vi "Practica3_led.vi"() -> ()   [LabVIEW 2015]
uses:
  <vilib>/LabVIEW Interface for Arduino/Type Defs/Pin Mode.ctl
  <vilib>/LabVIEW Interface for Arduino/LabVIEW Interface for Arduino.lvlib
panel:
  in  "Encendido":dbl format="%#.4g"
  in  "Apagado":dbl
  in  "stop":bool
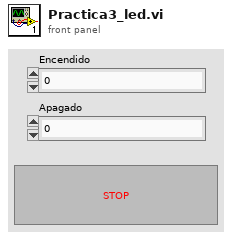
[diagram p1: front panel]
types:
  T1 = typedef "LabVIEW Interface for Arduino.lvlib/Pin Mode.ctl" = enum8{"Input", "Output"}
  T2 = typedef "LabVIEW Interface for Arduino.lvlib/Arduino Resource.ctl" = cluster{"VISA resource":refnum<visa-resource-name>, "Board Type":T3, "Connection Type":enum8{"USB / Serial"}, "Bytes Per Packet (15)":u8}
  T3 = typedef "LabVIEW Interface for Arduino.lvlib/Board Type.ctl" = enum16{"Uno", "Dimuelanove w/Atmega 328", "Mega 2560"}
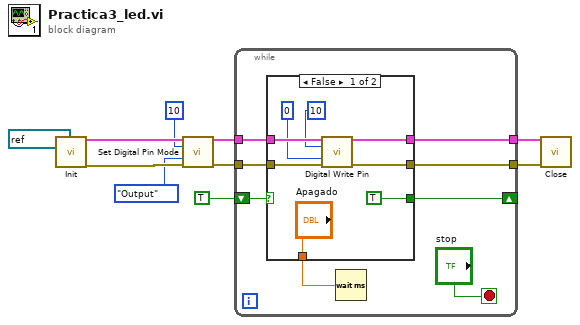
[diagram p0: block diagram]
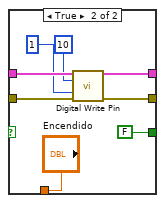
[diagram p2: hidden frame]
diagram:
  n1 = call <vilib>:"Init.vi"("VISA resource"=refnum<visa-resource-name> "COM4") -> ("Arduino Resource"=w9:T2, "error out"=w8:errorcluster)  [unwired: 17 in]
  n2 = call <vilib>:"Set Digital Pin Mode.vi"("Arduino Resource"=w9, "Digital I/O Pin"=u8 10, "Pin Mode (Input)"=Pin_Mode."Output", "error in"=w8) -> ("Arduino Resource"=w7:T2, "error out"=w6:errorcluster)  [unwired: 10 in]
  n3 = while {
    tunnel: w7 -> [w18]
    tunnel: w6 -> [w14]
    tunnel: [w16] -> w3
    tunnel: [w15] -> w2
    shift-right: [w12] -> _
    shift-left: TRUE -> [w11]
    stop <- "stop" stop-if-true
    n4 = case shown="False" w11 {
      tunnel: w18 -> [w24 w34]
      tunnel: [w26 w32] -> w16
      tunnel: [w25 w31] -> w15
      tunnel: w14 -> [w23 w30]
      tunnel: ["Apagado" "Encendido"] -> w13
      tunnel: [TRUE FALSE] -> w12
      frame False {
        n5 = call <vilib>:"Digital Write Pin.vi"("Arduino Resource"=w24, "Digital I/O Pin (0)"=u8 10, "Value (0)"=u8 0, "error in"=w23) -> ("Arduino Resource"=w26:T2, "error out"=w25:errorcluster)  [unwired: 10 in]
      }
      frame True {
        n6 = call <vilib>:"Digital Write Pin.vi"("Arduino Resource"=w34, "Digital I/O Pin (0)"=u8 10, "Value (0)"=u8 1, "error in"=w30) -> ("Arduino Resource"=w32:T2, "error out"=w31:errorcluster)  [unwired: 10 in]
      }
    }
    n7 = Wait (ms)(milliseconds to wait=w13) -> ()  [unwired: 1 out]
  }
  n8 = call <vilib>:"Close.vi"("Arduino Resource"=w3, "error in"=w2) -> ()  [unwired: 13 in, 1 out]
